vi "TopToCurrent.vi"(11 "States":cluster{"Current State":T1, "Next States":T2}) -> (3 "States":cluster{"Current State":T1, "Next States":T2})   [LabVIEW 2020]
uses:
  TDefs/State.ctl
  TDefs/States.ctl
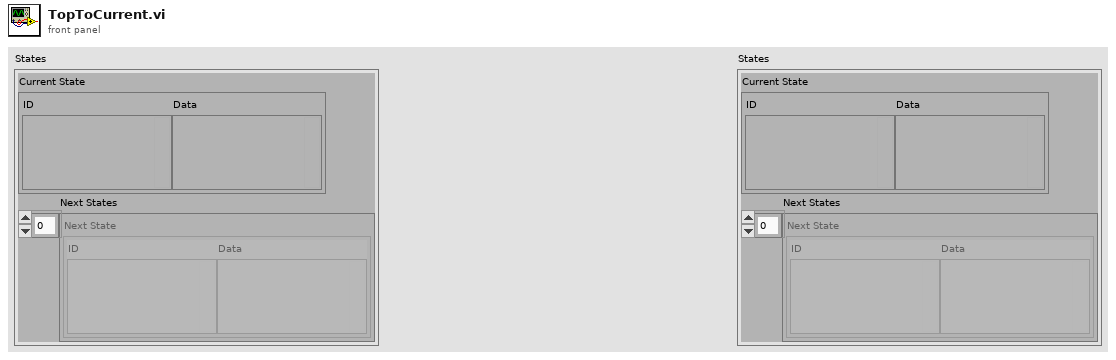
[diagram p1: front panel]
types:
  T1 = typedef "State.ctl" = cluster{"ID":variant, "Data":variant}
  T2 = typedef "States.ctl" = T1[]
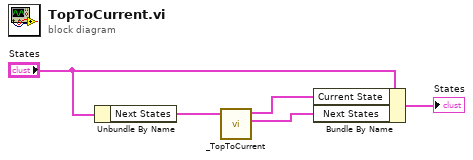
[diagram p0: block diagram]
diagram:
  n1 = Unbundle By Name("States") -> ("Next States"=w1:T2)
  n2 = call "_TopToCurrent.vi"("Next States in"=w1) -> ("Next States out"=w2:T2, "Next State"=w3:T1)  [unwired: 9 in]
  n3 = Bundle By Name(cluster="States", "Current State"=w3, "Next States"=w2) -> (→"States":cluster{"Current State":T1, "Next States":T2})
